vi "Dequeue Message.vi"(6 "timeout message (idle)":string="idle", 8 "error in (no error)":errorcluster, 9 "timeout in ms (-1)":i32, 11 "Message Queue":refnum<queue>) -> (0 "error out":errorcluster, 1 "Message Data":variant, 2 "Message":string, 3 "dup Message Queue":refnum<queue>)   [LabVIEW 2019, in "Message Queue.lvlib"]
doc: "This VI pulls messages off the Message Queue."
uses:
  Message Queue.lvlib
  Message Cluster.ctl
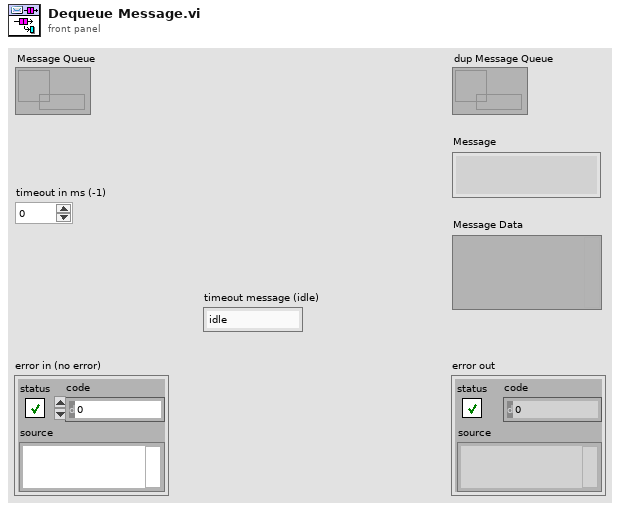
[diagram p1: front panel]
types:
  T1 = typedef "Message Queue.lvlib/Message Cluster.ctl" = cluster{"Message":string, "Message Data":variant}
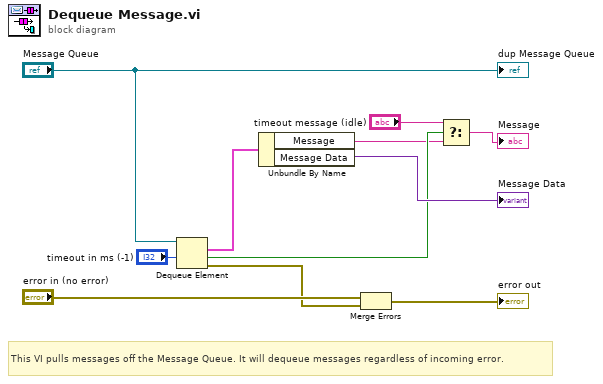
[diagram p0: block diagram]
diagram:
  # "This VI pulls messages off the Message Queue. It will dequeue messages regardless of incoming error."
  n1 = Dequeue Element(queue="Message Queue", timeout in ms (-1)="timeout in ms (-1)") -> (element=w9:T1, timed out?=w3:bool, error out=w6:errorcluster)  [unwired: 1 in, 1 out]
  n2 = Unbundle By Name(w9) -> ("Message"=w2:string, "Message Data"=→"Message Data":variant)
  n3 = Merge Errors("error in (no error)", w6) -> (→"error out":errorcluster)
  n4 = Select(t="timeout message (idle)", s=w3, f=w2) -> (s? t:f=→"Message":string)
  "dup Message Queue" <- "Message Queue"
